vi "MC-21C Driver_calculated.vi"(0 "Peristaltic Pump COM":refnum<visa-resource-name>="COM3", 1 "Speed (rpm)":string="20", 5 "Operation":T1(ring), 7 "Address":i16=1, 9 "Set address (0-255)":i16, 12 "Step":string="200") -> (6 "Current address":i32, 10 "Output string":string, 15 "Read string":string)   [LabVIEW 2023]
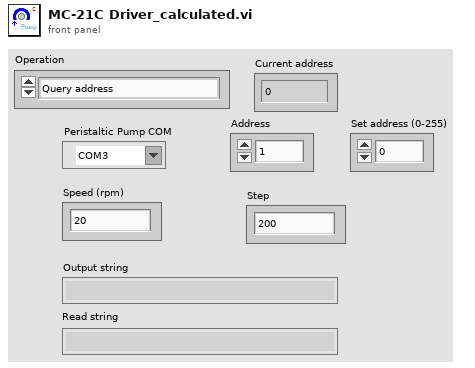
[diagram p1: front panel]
types:
  T1 = enum16{"Query address", "Set address", "Set speed", "Clockwise rotation", "Counterclockwise rotation", "Stop"}
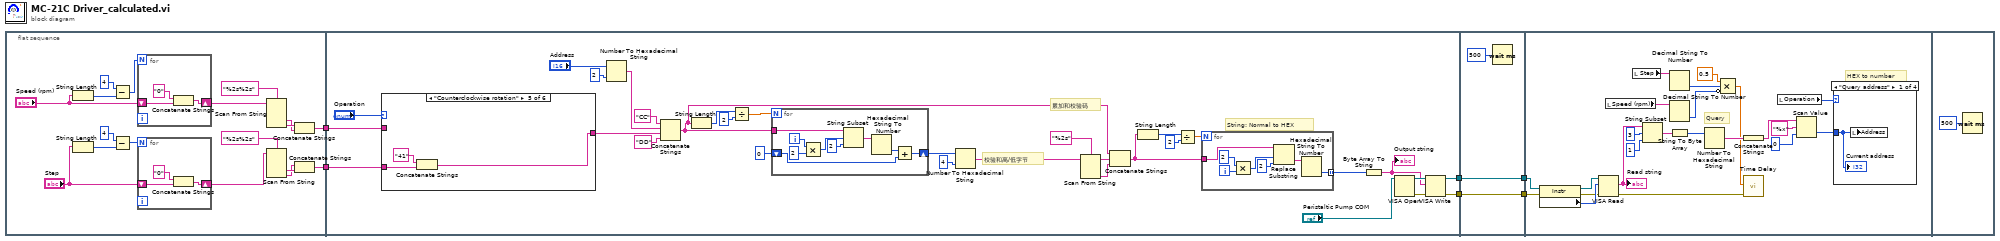
[diagram p0: block diagram]
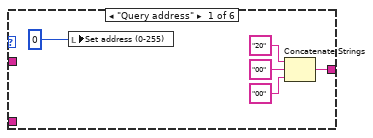
[diagram p2: hidden frame]
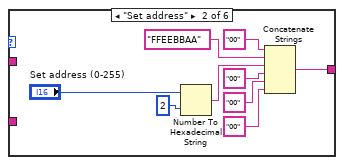
[diagram p3: hidden frame]
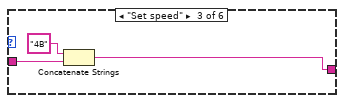
[diagram p4: hidden frame]
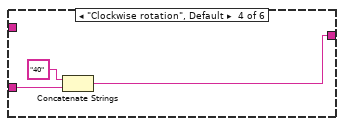
[diagram p5: hidden frame]
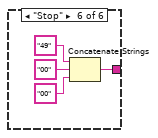
[diagram p6: hidden frame]
diagram:
  n1 = flat-sequence {
    tunnel: [w10] -> w2
    tunnel: [w9] -> w1
    tunnel: [w36] -> w6
    tunnel: [w35] -> w4
    tunnel: w2 -> [w33]
    tunnel: w1 -> [w32]
    tunnel: w6 -> [w107]
    tunnel: [w107] -> w5
    tunnel: w4 -> [w106]
    tunnel: [w106] -> w3
    tunnel: w5 -> [w127]
    tunnel: w3 -> [w126]
    frame #0 {
      n2 = String Length(string="Speed (rpm)") -> (length=w19:i32)
      n3 = String Length(string="Step") -> (length=w24:i32)
      n4 = Subtract(x=4, y=w19) -> (x-y=w21:i32)
      n5 = Subtract(x=4, y=w24) -> (x-y=w22:i32)
      n6 = for {
        N: w21 -> [_]
        shift-right: [w25] -> w11
        shift-left: "Speed (rpm)" -> [w27]
        n7 = Concatenate Strings("0" ("string"), w27) -> (w25:string)
      }
      n8 = for {
        N: w22 -> [_]
        shift-right: [w28] -> w18
        shift-left: "Step" -> [w30]
        n9 = Concatenate Strings("0" ("string"), w30) -> (w28:string)
      }
      n10 = Scan From String(format string="%2s%2s", input string=w11) -> (output 1=w13:string, output 2=w14:string)  [unwired: 4 in, 3 out]
      n11 = Scan From String(format string="%2s%2s", input string=w18) -> (output 1=w16:string, output 2=w15:string)  [unwired: 4 in, 3 out]
      n12 = Concatenate Strings(w14, w13) -> (w9:string)
      n13 = Concatenate Strings(w15, w16) -> (w10:string)
    }
    frame #1 {
      # "String: Normal to HEX"
      # "校验和高/低字节"
      # "累加和校验码"
      n14 = case shown="\"Counterclockwise rotation\"" "Operation" {
        tunnel: [w78 w83 w93 w96 w99 w101] -> w56
        tunnel: w33 -> [_ _ _ w95 w98 _]
        tunnel: w32 -> [_ _ w92 _ _ _]
        frame "Query address" {
          n15 = local write "Set address (0-255)"(i16 0 ("Address (0-255)")) -> ()
          n16 = Concatenate Strings("20" ("string"), "00" ("string"), "00" ("string")) -> (w78:string)
        }
        frame "Set address" {
          n17 = Number To Hexadecimal String(1:i16 2 ("width (-)"), 2:"Set address (0-255)") -> (0:w88:string)
          n18 = Concatenate Strings("00" ("string"), "FFEEBBAA" ("string"), w88, "00" ("string"), "00" ("string"), "00" ("string")) -> (w83:string)
        }
        frame "Set speed" {
          n19 = Concatenate Strings("4B" ("string"), w92) -> (w93:string)
        }
        frame "Clockwise rotation", Default {
          n20 = Concatenate Strings("40" ("string"), w95) -> (w96:string)
        }
        frame "Counterclockwise rotation" {
          n21 = Concatenate Strings("41" ("string"), w98) -> (w99:string)
        }
        frame "Stop" {
          n22 = Concatenate Strings("49" ("string"), "00" ("string"), "00" ("string")) -> (w101:string)
        }
      }
      n23 = Number To Hexadecimal String(1:i16 2 ("width (-)"), 2:"Address") -> (0:w59:string)
      n24 = Concatenate Strings("CC" ("string"), w59, w56, "DD" ("string")) -> (w47:string)
      n25 = String Length(string=w47) -> (length=w55:i32)
      n26 = Divide(x=w55, y=2) -> (x/y=w53:dbl)
      n27 = for {
        N: w53 -> [_]
        shift-right: [w69] -> w51
        shift-left: 0 ("length (rest)") -> [w70]
        tunnel: w47 -> [w77]
        i -> [w74]
        n28 = Multiply(x=w74, y=2) -> (x*y=w73:i32)
        n29 = String Subset(string=w77, offset (0)=w73, length (rest)=2 ("length (rest)")) -> (substring=w72:string)
        n30 = Hexadecimal String To Number(string=w72) -> (number=w71:u32)  [unwired: 2 in, 1 out]
        n31 = Add(x=w71, y=w70) -> (x+y=w69:u32)
      }
      n32 = Number To Hexadecimal String(1:i16 4 ("width (-)"), 2:w51) -> (0:w49:string)
      n33 = Scan From String(format string="%2s", input string=w49) -> (remaining string=w46:string, output 1=w45:string)  [unwired: 3 in, 2 out]
      n34 = Concatenate Strings(w47, w46, w45) -> (w38:string)
      n35 = String Length(string=w38) -> (length=w41:i32)
      n36 = Divide(x=w41, y=2) -> (x/y=w40:dbl)
      n37 = for {
        N: w40 -> [_]
        tunnel: w38 -> [w68]
        tunnel: [w62] -> w42 mode=indexing
        i -> [w67]
        n38 = Multiply(x=2, y=w67) -> (x*y=w65:i32)
        n39 = Replace Substring(2:2 ("长度（子字符串长度）"), 3:w65, 5:w68) -> (0:w63:string)  [unwired: 1 in, 1 out]
        n40 = Hexadecimal String To Number(string=w63) -> (number=w62:u32)  [unwired: 2 in, 1 out]
      }
      n41 = Byte Array To String(unsigned byte array=w42) -> (string=w34:string)
      "Output string" <- w34
      n42 = VISA Open(VISA resource name="Peristaltic Pump COM") -> (VISA resource name=w44:refnum<visa-resource-name>, error out=w43:errorcluster)  [unwired: 4 in]
      n43 = VISA Write(VISA resource name=w44, write buffer=w34, error in (no error)=w43) -> (VISA resource name out=w36:refnum<visa-resource-name>, error out=w35:errorcluster)  [unwired: 1 out]
    }
    frame #2 {
      n44 = Wait (ms)(milliseconds to wait=u32 500) -> ()  [unwired: 1 out]
    }
    frame #3 {
      # "HEX to number"
      # "Query"
      n45 = property class="Instr"(reference=w127, error in=w126) -> (reference out=w128:refnum<visa-resource-name>, error out=w129:errorcluster, "Serial Settings:Number of Bytes at Serial Port"=w130:u32)
      n46 = VISA Read(VISA resource name=w128, byte count=w130, error in (no error)=w129) -> (read buffer=w125:string, error out=w114:errorcluster)  [unwired: 2 out]
      "Read string" <- w125
      n47 = local read "Speed (rpm)"() -> (w112:string)
      n48 = local read "Step"() -> (w113:string)
      n49 = String Subset(string=w125, offset (0)=3, length (rest)=1 ("length (rest)")) -> (substring=w118:string)
      n50 = Decimal String To Number(string=w113) -> (number=w111:i32)  [unwired: 2 in, 1 out]
      n51 = Decimal String To Number(string=w112) -> (number=w110:i32)  [unwired: 2 in, 1 out]
      n52 = String To Byte Array(string=w118) -> (unsigned byte array=w120:u8[])
      n53 = Number To Hexadecimal String(2:w120) -> (0:w119:string[])  [unwired: 1 in]
      n54 = Compound Arithmetic op=MULTIPLY(0.5 ("value"), w111, invert w110) -> (w108:dbl)
      n55 = Concatenate Strings(w119) -> (w117:string)
      n56 = call "Time Delay"("error in (no error)"=w114, "Delay Time (s)"=w108) -> ()  [unwired: 9 in, 1 out]
      n57 = local read "Operation"() -> (w115:T1)
      n58 = Scan Value(string=w117, format string="%x", default (0 dbl)=0 ("length (rest)")) -> (value=w116:i32)  [unwired: 1 out]
      n59 = case shown="\"Query address\"" w115 {
        tunnel: w116 -> [w131 _ _ _]
        frame "Query address" {
          n60 = local write "Address"(w131) -> ()
          "Current address" <- w131
        }
        frame "Clockwise rotation" {
        }
        frame "Counterclockwise rotation" {
        }
        frame "Stop", Default {
        }
      }
    }
    frame #4 {
      n61 = Wait (ms)(milliseconds to wait=u32 500) -> ()  [unwired: 1 out]
    }
  }
